vi "Phasor Subtract Baseline from Array [DBL].vi"(0 "X Array":dbl[](array[numeric]), 1 "Method (Min)":T1=enum."Min", 2 "Gate Duration":dbl[unit]=nan, 3 "Laser Period":dbl[unit]=nan, 5 "Y Array":dbl[](array[numeric]), 7 "Max X":dbl=nan, 9 "Min X":dbl=nan, 11 "Error In":errorcluster, 12 "Background Constant":dbl) -> (4 "Bkgd-subtracted Y Array":dbl[](array[numeric]), 6 "Background/Gate":dbl, 8 "Lifetime":dbl[unit]=nan, 10 "Bkgd-subtracted Intensity (theo)":dbl, 14 "Message":string, 15 "Error Out":errorcluster)   [LabVIEW 2021, in "Phasor.lvlib"]
uses:
  Phasor.lvlib
  AlliGator/Decay Analysis/Decay Preprocessing/AlliGator Baseline Subtraction Method.ctl
  <vilib>/Utility/error.llb/Error Cluster From Error Code.vi
  <vilib>/ErrorRing/Error Ring.xnode
  Comparison/Comparison.lvlib
  AlliGator/Decay Analysis/Decay Preprocessing/AlliGator Decay Preprocessing.lvlib
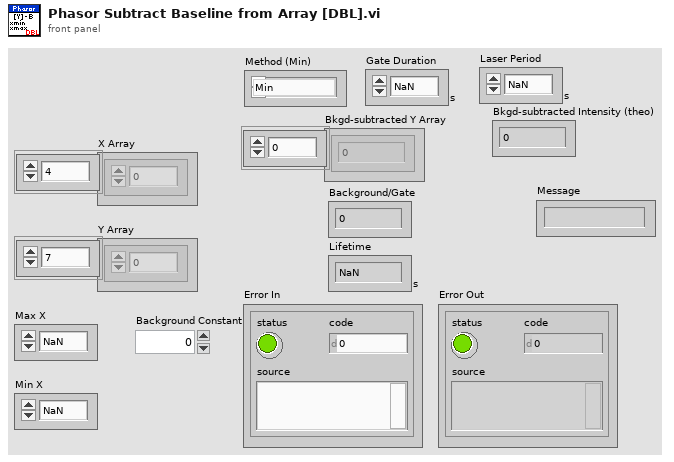
[diagram p1: front panel]
types:
  T1 = typedef "AlliGator Decay Preprocessing.lvlib/AlliGator Baseline Subtraction Method.ctl" = enum16{"Mean", "Min", "Square Gated Single-Exponential", "File", "Constant"}
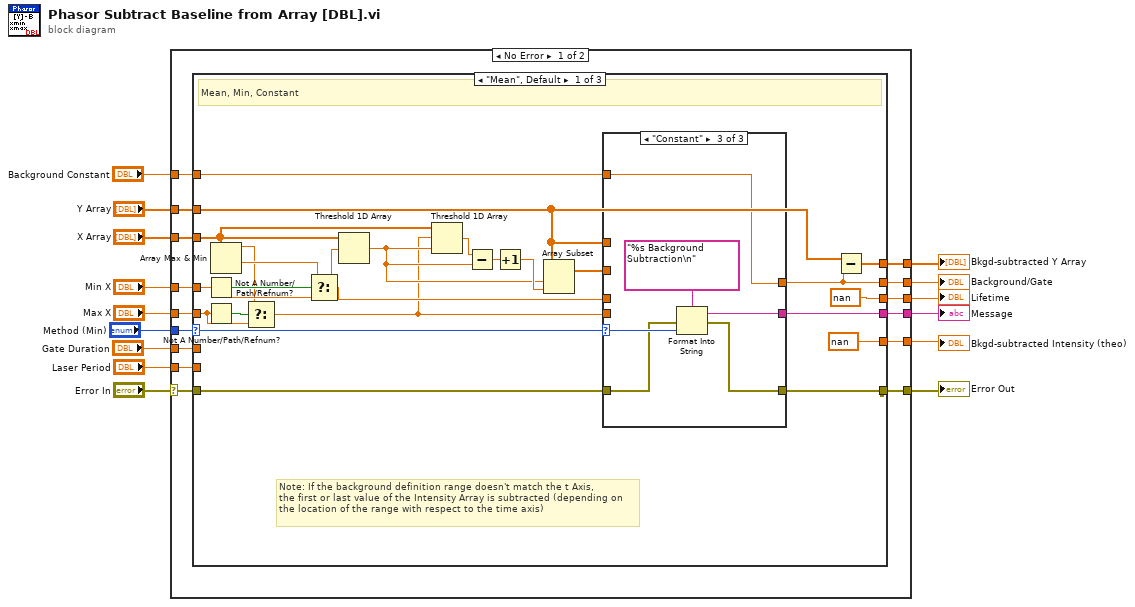
[diagram p0: block diagram]
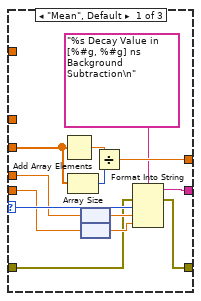
[diagram p2: hidden frame]
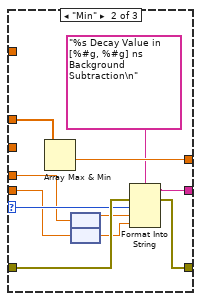
[diagram p3: hidden frame]
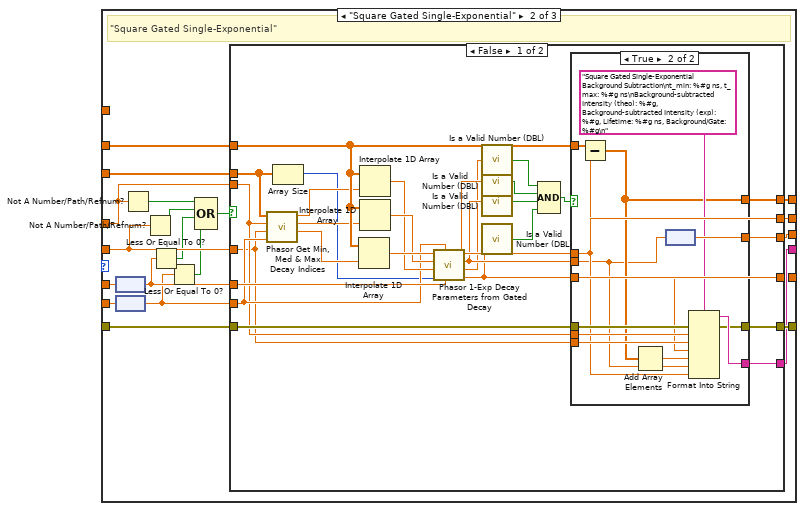
[diagram p4: hidden frame]
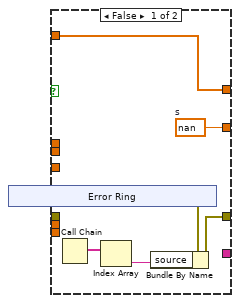
[diagram p5: hidden frame]
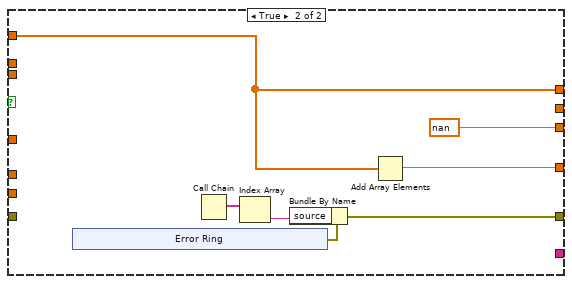
[diagram p6: hidden frame]
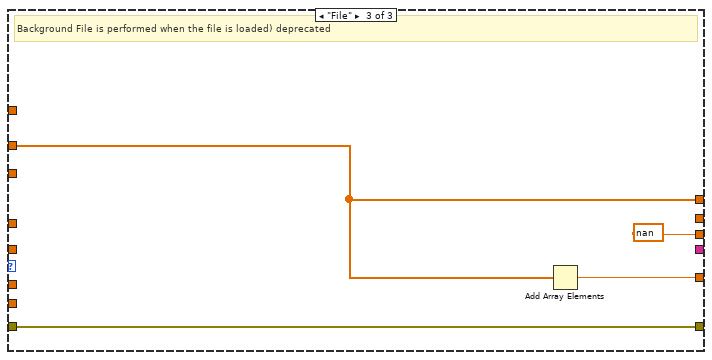
[diagram p7: hidden frame]
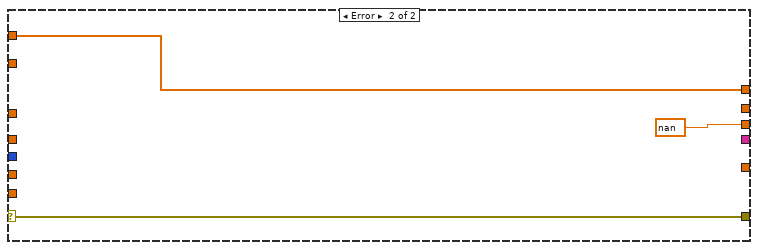
[diagram p8: hidden frame]
diagram:
  n1 = case shown="No Error" "Error In" {
    selector: "Error In" -> [w20 w172]
    tunnel: "Min X" -> [w30 _]
    tunnel: "Max X" -> [w29 _]
    tunnel: [w28 w170] -> w13
    tunnel: "X Array" -> [w27 _]
    tunnel: [w26 _] -> w11
    tunnel: "Y Array" -> [w25 w170]
    tunnel: "Method (Min)" -> [w24 _]
    tunnel: "Gate Duration" -> [w23 _]
    tunnel: "Laser Period" -> [w22 _]
    tunnel: [w21 dbl[unit] nan ("B")] -> w6
    tunnel: [w19 w172] -> w4
    tunnel: [w18 _] -> w3
    tunnel: [w17 _] -> w2
    tunnel: "Background Constant" -> [w16 _]
    frame No Error {
      n2 = case shown="\"Mean\", Default" w24 {
        selector: w24 -> [w40 _ _]
        tunnel: w27 -> [w47 w94 _]
        tunnel: [w39 w97 w167] -> w28
        tunnel: [w41 w104 _] -> w26
        tunnel: w25 -> [w37 w98 w167]
        tunnel: w29 -> [w44 w92 _]
        tunnel: w30 -> [w46 w95 _]
        tunnel: w23 -> [_ w102 _]
        tunnel: w22 -> [_ w91 _]
        tunnel: [dbl[unit] nan ("B") w103 dbl[unit] nan ("B")] -> w21
        tunnel: w20 -> [w32 w96 w168]
        tunnel: [w31 w93 w168] -> w19
        tunnel: [w33 w90 _] -> w18
        tunnel: [nan ("I") w89 w166] -> w17
        tunnel: w16 -> [w36 _ _]
        frame "Mean", Default {
          # "Note: If the background definition range doesn't match the t Axis,\nthe first or last value of the Intensity Array is subtracted (depending on the location of the range with respect to the time axis)"
          # "Mean, Min, Constant"
          n3 = Not A Number/Path/Refnum?(number/path/refnum=w46) -> (NaN/Path/Refnum?=w49:bool)
          n4 = Not A Number/Path/Refnum?(number/path/refnum=w44) -> (NaN/Path/Refnum?=w48:bool)
          n5 = Array Max & Min(array=w47) -> (max value=w43:dbl, min value=w45:dbl)  [unwired: 2 out]
          n6 = Select(t=w43, s=w48, f=w44) -> (s? t:f=w34:dbl)
          n7 = Select(t=w45, s=w49, f=w46) -> (s? t:f=w35:dbl)
          n8 = Threshold 1D Array(2:w35, 3:w47) -> (0:w50:dbl)  [unwired: 1 in]
          n9 = Threshold 1D Array(1:w50, 2:w34, 3:w47) -> (0:w54:dbl)
          n10 = Subtract(x=w54, y=w50) -> (x-y=w53:dbl)
          n11 = Increment(x=w53) -> (x+1=w51:dbl)
          n12 = Array Subset(array=w37, index=w50, length=w51) -> (w52:dbl[])
          n13 = case shown="\"Constant\"" w40 {
            selector: w40 -> [w62 w74 w83]
            tunnel: w52 -> [w65 _ _]
            tunnel: [w66 w78 w84] -> w41
            tunnel: w37 -> [_ w77 _]
            tunnel: w36 -> [_ _ w84]
            tunnel: [w55 w68 w79] -> w33
            tunnel: w35 -> [w61 w71 _]
            tunnel: w34 -> [w59 w70 _]
            tunnel: w32 -> [w57 w76 w81]
            tunnel: [w56 w75 w80] -> w31
            frame "Mean", Default {
              n14 = Add Array Elements(numeric array=w65) -> (sum=w67:dbl)
              n15 = Array Size(array=w65) -> (size(s)=w64:i32)
              n16 = node(w61) -> (w60:dbl[unit])
              n17 = node(w59) -> (w58:dbl[unit])
              n18 = Divide(x=w67, y=w64) -> (x/y=w66:dbl)
              n19 = Format Into String(format string="%s Decay Value in [%#g, %#g] ns Background Subtraction\n", error in=w57, w62, w60, w58) -> (resulting string=w55:string, error out=w56:errorcluster)  [unwired: 1 in]
            }
            frame "Min" {
              n20 = Array Max & Min(array=w77) -> (min value=w78:dbl)  [unwired: 3 out]
              n21 = node(w71) -> (w73:dbl[unit])
              n22 = node(w70) -> (w72:dbl[unit])
              n23 = Format Into String(format string="%s Decay Value in [%#g, %#g] ns Background Subtraction\n", error in=w76, w74, w73, w72) -> (resulting string=w68:string, error out=w75:errorcluster)  [unwired: 1 in]
            }
            frame "Constant" {
              n24 = Format Into String(format string="%s Background Subtraction\n", error in=w81, w83) -> (resulting string=w79:string, error out=w80:errorcluster)  [unwired: 1 in]
            }
          }
          n25 = Subtract(x=w37, y=w41) -> (x-y=w39:dbl[])
        }
        frame "Square Gated Single-Exponential" {
          # "\"Square Gated Single-Exponential\""
          n26 = node(w102) -> (w87:dbl)
          n27 = node(w91) -> (w86:dbl)
          n28 = Not A Number/Path/Refnum?(number/path/refnum=w95) -> (NaN/Path/Refnum?=w101:bool)
          n29 = Not A Number/Path/Refnum?(number/path/refnum=w92) -> (NaN/Path/Refnum?=w100:bool)
          n30 = Less Or Equal To 0?(x=w87) -> (x <= 0?=w88:bool)
          n31 = Less Or Equal To 0?(x=w86) -> (x <= 0?=w85:bool)
          n32 = Compound Arithmetic op=OR(w101, w100, w88, w85) -> (w99:bool)
          n33 = case shown="False" w99 {
            tunnel: [w113 _] -> w104
            tunnel: [w131 dbl[unit] nan ("B")] -> w103
            tunnel: w87 -> [w126 _]
            tunnel: w98 -> [w130 w160]
            tunnel: [w114 w160] -> w97
            tunnel: w96 -> [w119 _]
            tunnel: w95 -> [w118 _]
            tunnel: w94 -> [w116 _]
            tunnel: [w120 w155] -> w93
            tunnel: w92 -> [w117 _]
            tunnel: w86 -> [w125 _]
            tunnel: [w121 _] -> w90
            tunnel: [w111 w159] -> w89
            frame False {
              n34 = call "Phasor Get Min, Med & Max Decay Indices.vi"("Period"=w125, "Max X"=w117, "Min X"=w118, "X Array"=w116) -> ("Max X idx"=w122:dbl, "Med X idx"=w123:dbl, "Min X idx"=w124:dbl)  [unwired: 5 in]
              n35 = Array Size(array=w116) -> (size(s)=w115:i32)
              n36 = Interpolate 1D Array(1:w122, 2:w130) -> (0:w129:dbl)
              n37 = Interpolate 1D Array(1:w124, 2:w130) -> (0:w127:dbl)
              n38 = Interpolate 1D Array(1:w123, 2:w130) -> (0:w128:dbl)
              n39 = call "Phasor 1-Exp Decay Parameters from Gated Decay.vi"("Gate Width: W"=w126, "period: T"=w125, "# Gates"=w115, "Min Decay"=w127, "Mid Decay"=w128, "Max Decay"=w129) -> ("I"=w111:dbl, "x"=w105:dbl, "tau"=w112:dbl, "B"=w113:dbl)  [unwired: 2 in]
              n40 = call "Is a Valid Number (DBL).vi"("Number"=w105) -> ("Valid Number?"=w110:bool)  [unwired: 8 in]
              n41 = call "Is a Valid Number (DBL).vi"("Number"=w113) -> ("Valid Number?"=w109:bool)  [unwired: 8 in]
              n42 = call "Is a Valid Number (DBL).vi"("Number"=w112) -> ("Valid Number?"=w108:bool)  [unwired: 8 in]
              n43 = call "Is a Valid Number (DBL).vi"("Number"=w111) -> ("Valid Number?"=w107:bool)  [unwired: 8 in]
              n44 = Compound Arithmetic op=AND(w110, w109, w108, w107) -> (w106:bool)
              n45 = case shown="True" w106 {
                tunnel: [w136 w154] -> w131
                tunnel: w130 -> [w137 w153]
                tunnel: [_ w152] -> w121
                tunnel: [w134 w151] -> w120
                tunnel: w119 -> [_ w150]
                tunnel: w118 -> [_ w148]
                tunnel: w117 -> [_ w147]
                tunnel: [w137 w146] -> w114
                tunnel: w113 -> [_ w144]
                tunnel: w112 -> [_ w143]
                tunnel: w111 -> [_ w142]
                frame False {
                  w136 = dbl[unit] nan  # s
                  n46 = xnode "Error Ring"() -> ("error out"=w135:errorcluster)
                  n47 = Call Chain() -> (call chain=w133:string[])
                  n48 = Index Array(array=w133) -> (element=w132:string)  [unwired: 1 in]
                  n49 = Bundle By Name(cluster=w135, "source"=w132) -> (w134:errorcluster)
                }
                frame True {
                  n50 = Subtract(x=w153, y=w144) -> (x-y=w146:dbl[])
                  n51 = Add Array Elements(numeric array=w146) -> (sum=w145:dbl)
                  n52 = node(w143) -> (w154:dbl[unit])
                  n53 = Format Into String(format string="Square Gated Single-Exponential Background Subtraction\nt_min: %#g ns, t_max: %#g ns\nBackground-subtracted Intensity (theo): %#g, Background-subtracted Intensity (exp): %#g, Lifetime: %#g ns, Background/Gate: %#g\n", error in=w150, w148, w147, w142, w145, w143, w144) -> (resulting string=w152:string, error out=w151:errorcluster)  [unwired: 1 in]
                }
              }
            }
            frame True {
              n54 = xnode "Error Ring"() -> ("error out"=w156:errorcluster)
              n55 = Call Chain() -> (call chain=w158:string[])
              n56 = Index Array(array=w158) -> (element=w157:string)  [unwired: 1 in]
              n57 = Bundle By Name(cluster=w156, "source"=w157) -> (w155:errorcluster)
              n58 = Add Array Elements(numeric array=w160) -> (sum=w159:dbl)
            }
          }
        }
        frame "File" {
          # "Background File is performed when the file is loaded) deprecated"
          n59 = Add Array Elements(numeric array=w167) -> (sum=w166:dbl)
        }
      }
    }
    frame Error {
    }
  }
  "Bkgd-subtracted Y Array" <- w13
  "Background/Gate" <- w11
  "Error Out" <- w4
  "Lifetime" <- w6
  "Message" <- w3
  "Bkgd-subtracted Intensity (theo)" <- w2
